vi "Setting Custom Tree Item Symbols.vi"() -> ()   [LabVIEW 2023]
doc: "This example shows how to replace item symbols in a tree control with custom item symbols."
panel:
  in  "Tree":string(tree)
  # "Overview: Demonstrates how to replace item symbols in a Tree Control with custom item symbols.\nInstructions:\nRun the VI. The VI replaces all instances of the empty diamond symbol with a custom item symbol."
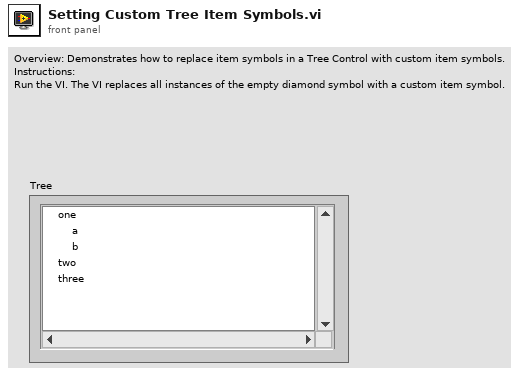
[diagram p1: front panel]
types:
  T1 = typedef "imagedata.ctl" = cluster{"image type":i32, "image depth":i32, "image":u8[], "mask":u8[], "colors":u32[], "Rectangle":cluster{"left":i16, "top":i16, "right":i16, "bottom":i16}}
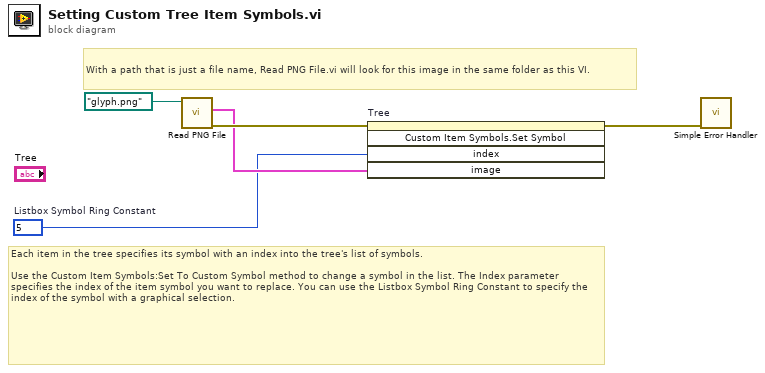
[diagram p0: block diagram]
diagram:
  w2 = 5  # Listbox Symbol Ring Constant
  # "With a path that is just a file name, Read PNG File.vi will look for this image in the same folder as this VI."
  # "Each item in the tree specifies its symbol with an index into the tree's list of symbols.\n\nUse the Custom Item Symbols:Set To Custom Symbol method to change a symbol in the list. The Index parameter specifies the index of the item symbol you want to replace. You can use the Listbox Symbol Ring Constant to specify the index of the symbol with a graphical selection."
  n1 = call <vilib>:"Read PNG File.vi"("path to PNG file"=path "glyph.png" ("Path to PNG file for symbol")) -> ("error out"=w5:errorcluster, "image data"=w3:T1)  [unwired: 8 in, 1 out]
  n2 = invoke on="Tree" class="TreeControl (strict)" method="Custom Item Symbols.Set Symbol"(error in=w5, "index"=w2, "image"=w3) -> (error out=w1:errorcluster)  [unwired: 2 in, 4 out]
  n3 = call <vilib>:"Simple Error Handler.vi"("error in (no error)"=w1) -> ()  [unwired: 4 in, 5 out]
